vi "convertXMLStringToDBL.vi"(7 "DataType":dbl, 8 "error in (no error)":errorcluster, 10 "XMLContents In":string) -> (0 "error out":errorcluster, 2 "DBL Out":dbl)   [LabVIEW 2012, in "XMLStringToDataConverter.lvlib"]
uses:
  <userlib>/Common/XML/XMLStringToDataConverter/XMLStringToDataConverter.lvlib
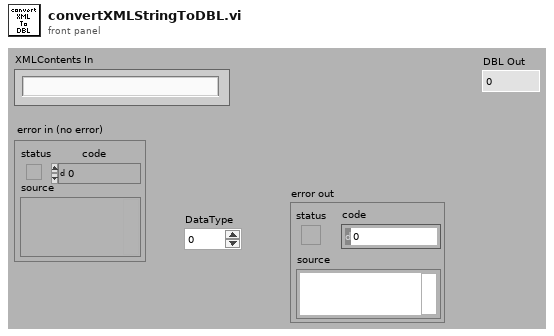
[diagram p1: front panel]
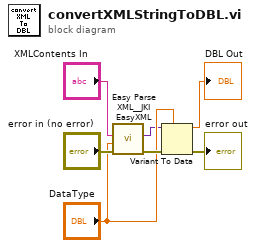
[diagram p0: block diagram]
diagram:
  n1 = call <vilib>:"Easy Parse XML__JKI EasyXML.vi"("error in (no error)"="error in (no error)", "LabVIEW Data (Type)"="DataType", "XML String"="XMLContents In") -> ("error out"=w6:errorcluster, "LabVIEW Data"=w1:variant)  [unwired: 7 in]
  n2 = Variant To Data(error in=w6, type="DataType", Variant=w1) -> (data=→"DBL Out":dbl, error out=→"error out":errorcluster)
